vi "smart in(de) crement (SubVI).vi"(5 "upper limit in":i32, 7 "lower limit":i32, 8 "previous object":bool, 9 "next object":bool, 11 "Object":i32) -> (3 "Object out":i32)   [LabVIEW 2020]
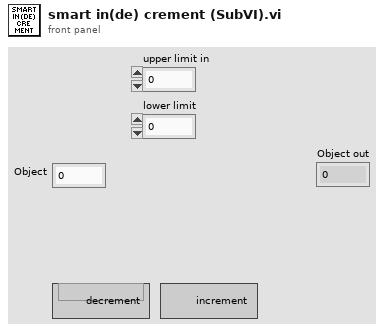
[diagram p1: front panel]
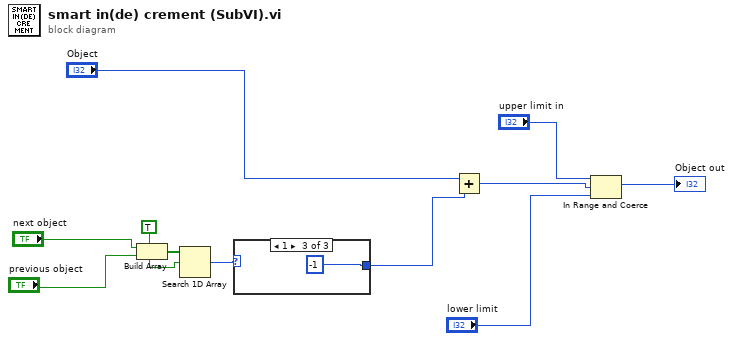
[diagram p0: block diagram]
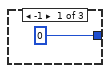
[diagram p2: hidden frame]
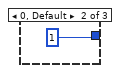
[diagram p3: hidden frame]
diagram:
  n1 = Build Array("next object", "previous object") -> (w1:bool[])
  n2 = Search 1D Array(1D array=w1, element=TRUE) -> (index of element=w3:i32)  [unwired: 1 in]
  n3 = case shown="1" w3 {
    tunnel: [0 ("lower limit") 1 ("y") -1 ("y")] -> w4
    frame -1 {
    }
    frame 0, Default {
    }
    frame 1 {
    }
  }
  n4 = Add(x="Object", y=w4) -> (x+y=w8:i32)
  n5 = In Range and Coerce(upper limit="upper limit in", x=w8, lower limit="lower limit") -> (coerced(x)=→"Object out":i32)  [unwired: 1 out]
